vi "sync init timing.vi"(8 "error in (no error)":errorcluster, 9 "data dictionary in":refnum<class "data dictionary.lvclass">, 10 "pointer in":u64, 11 "publish timing?":bool) -> (0 "error out":errorcluster, 2 "pointer out":u64, 3 "timing pointers":T2, 5 "timing indices":T1)   [LabVIEW 2014, in "Shared Memory runtime.lvclass"]
uses:
  Shared Memory runtime.lvclass
  <vilib>/NI/Tag Bus/dictionary/data dictionary.lvclass
  controls/sync timing pointers.ctl
  controls/sync timing indices.ctl
  <vilib>/NI/Tag Bus/tag/tag descriptor.lvclass/tag descriptor.ctl
  <vilib>/NI/Tag Bus/tag/read tag name.vi
  <vilib>/NI/Tag Bus/tag/read data type.vi
  <vilib>/NI/Tag Bus/dictionary/locate tag.vi
  configuration/Shared Memory configuration.lvclass
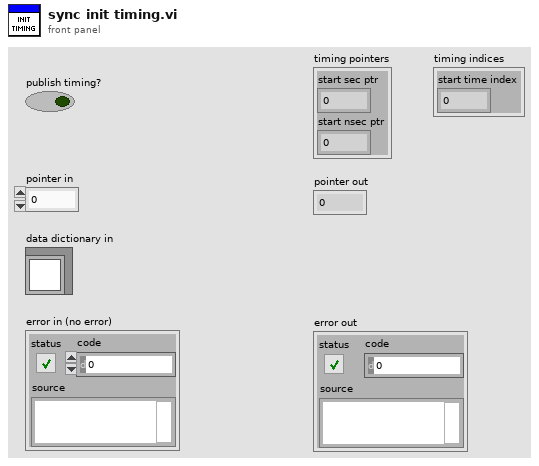
[diagram p1: front panel]
types:
  T1 = typedef "Shared Memory runtime.lvclass/sync timing indices.ctl" = cluster{"start time index":i32}
  T2 = typedef "Shared Memory runtime.lvclass/sync timing pointers.ctl" = cluster{"start sec ptr":u64, "start nsec ptr":u64}
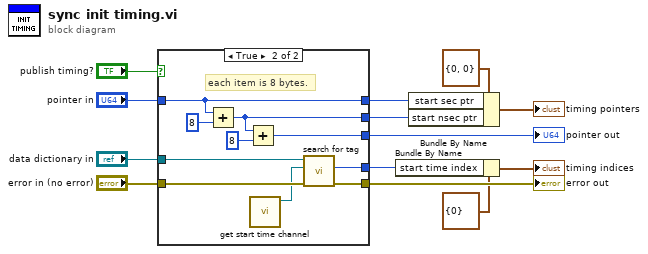
[diagram p0: block diagram]
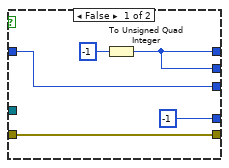
[diagram p2: hidden frame]
diagram:
  n1 = case shown="True" "publish timing?" {
    tunnel: "error in (no error)" -> [w17 w28]
    tunnel: "pointer in" -> [w18 w23]
    tunnel: [w15 w23] -> w8
    tunnel: [w15 w26] -> w9
    tunnel: [w18 w25] -> w3
    tunnel: [w17 w21] -> w4
    tunnel: "data dictionary in" -> [_ w22]
    tunnel: [-1 ("index") w20] -> w13
    frame False {
      n2 = To Unsigned Quad Integer(1:i64 -1) -> (0:w15:u64)
    }
    frame True {
      # "each item is 8 bytes."
      n3 = Add(x=w23, y=u64 8) -> (x+y=w26:u64)
      n4 = Add(x=w26, y=u64 8) -> (x+y=w25:u64)
      n5 = call "get start time channel.vi"() -> ("channel"=w19:refnum<class "TBM channel.lvclass">)  [unwired: 11 in]
      n6 = call <vilib>:"search for tag.vi"("error in"=w28, "system tag"=w19, "data dictionary in"=w22) -> ("error out"=w21:errorcluster, "index"=w20:i32)  [unwired: 6 in, 1 out]
    }
  }
  "error out" <- w4
  "pointer out" <- w3
  n7 = Bundle By Name(cluster=T1 {"start time index"=0} ("timing indices"), "start time index"=w13) -> (→"timing indices":T1)
  n8 = Bundle By Name(cluster=T2 {"start sec ptr"=0, "start nsec ptr"=0} ("timing pointers"), "start sec ptr"=w8, "start nsec ptr"=w9) -> (→"timing pointers":T2)
